vi "Phasor Index To String.vi"(11 "Phasor Index":i32) -> (3 "String":string)   [LabVIEW 2017, in "PMU Recorder Light.lvlib" / "Statnett C37.118 DLL.lvclass"]
uses:
  Statnett C37.118 DLL.lvclass
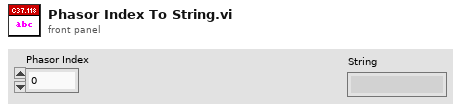
[diagram p1: front panel]
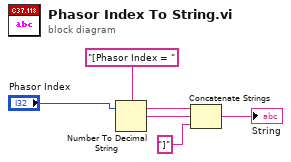
[diagram p0: block diagram]
diagram:
  n1 = Number To Decimal String(number="Phasor Index") -> (decimal integer string=w5:string)  [unwired: 1 in]
  n2 = Concatenate Strings("[Phasor Index = " ("string"), w5, "]" ("string")) -> (→"String":string)
